vi "9940 Pending IResponses is null--error.vi"(8 "error in":errorcluster, 11 "Argument":string) -> (0 "error out":errorcluster, 2 "Error Code":i32)   [LabVIEW 2020, in "CANopen.lvlib" / "Response Matcher.lvclass"]
uses:
  Response Matcher.lvclass
  Response Matcher.lvclass/Response Matcher.ctl
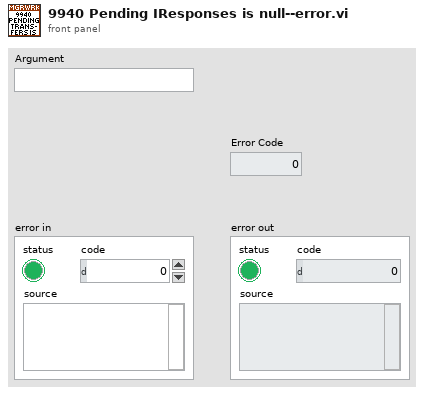
[diagram p1: front panel]
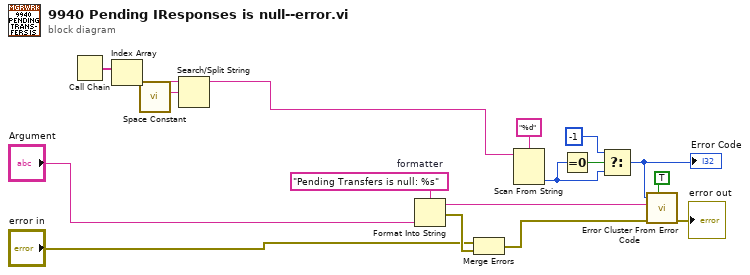
[diagram p0: block diagram]
diagram:
  w14 = "Pending Transfers is null: %s"  # formatter
  n1 = Call Chain() -> (call chain=w8:string[])
  n2 = Index Array(array=w8) -> (element=w12:string)  [unwired: 1 in]
  n3 = call <vilib>:"Space Constant.vi"() -> ("String"=w2:string)
  n4 = Search/Split String(string=w12, search string/char (-)=w2) -> (substring before match=w1:string)  [unwired: 1 in, 2 out]
  n5 = Format Into String(format string=w14, "Argument") -> (resulting string=w15:string, error out=w6:errorcluster)  [unwired: 2 in]
  n6 = Merge Errors("error in", w6) -> (w4:errorcluster)
  n7 = Scan From String(format string="%d", input string=w1) -> (output 1=w10:i32)  [unwired: 3 in, 3 out]
  n8 = Equal To 0?(x=w10) -> (x = 0?=w11:bool)
  n9 = Select(t=-1, s=w11, f=w10) -> (s? t:f=w7:i32)
  "Error Code" <- w7
  n10 = call <vilib>:"Error Cluster From Error Code.vi"("show call chain? (False)"=TRUE, "error in (no error)"=w4, "error message (\"\")"=w15, "error code (0)"=w7) -> ("error out"=→"error out":errorcluster)  [unwired: 5 in]
